vi "Logger.vi"(3 "Error In":errorcluster, 4 "Pipeline In":refnum<queue>, 5 "Logger Queue In":refnum<queue>) -> (0 "Error Out":errorcluster)   [LabVIEW 2016]
uses:
  Message Format.ctl
  StateDef_logger.ctl
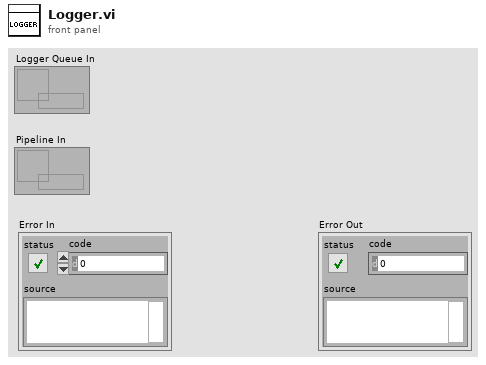
[diagram p1: front panel]
types:
  T1 = typedef "StateDef_Logger.ctl" = enum16{"Idle", "Open File", "Write to File", "Close File", "Exit"}
  T2 = enum16{"open", "open or create", "create or replace", "create", "open (read-only)"}
  T3 = typedef "Message Format.ctl" = cluster{"header":string, "data":variant}
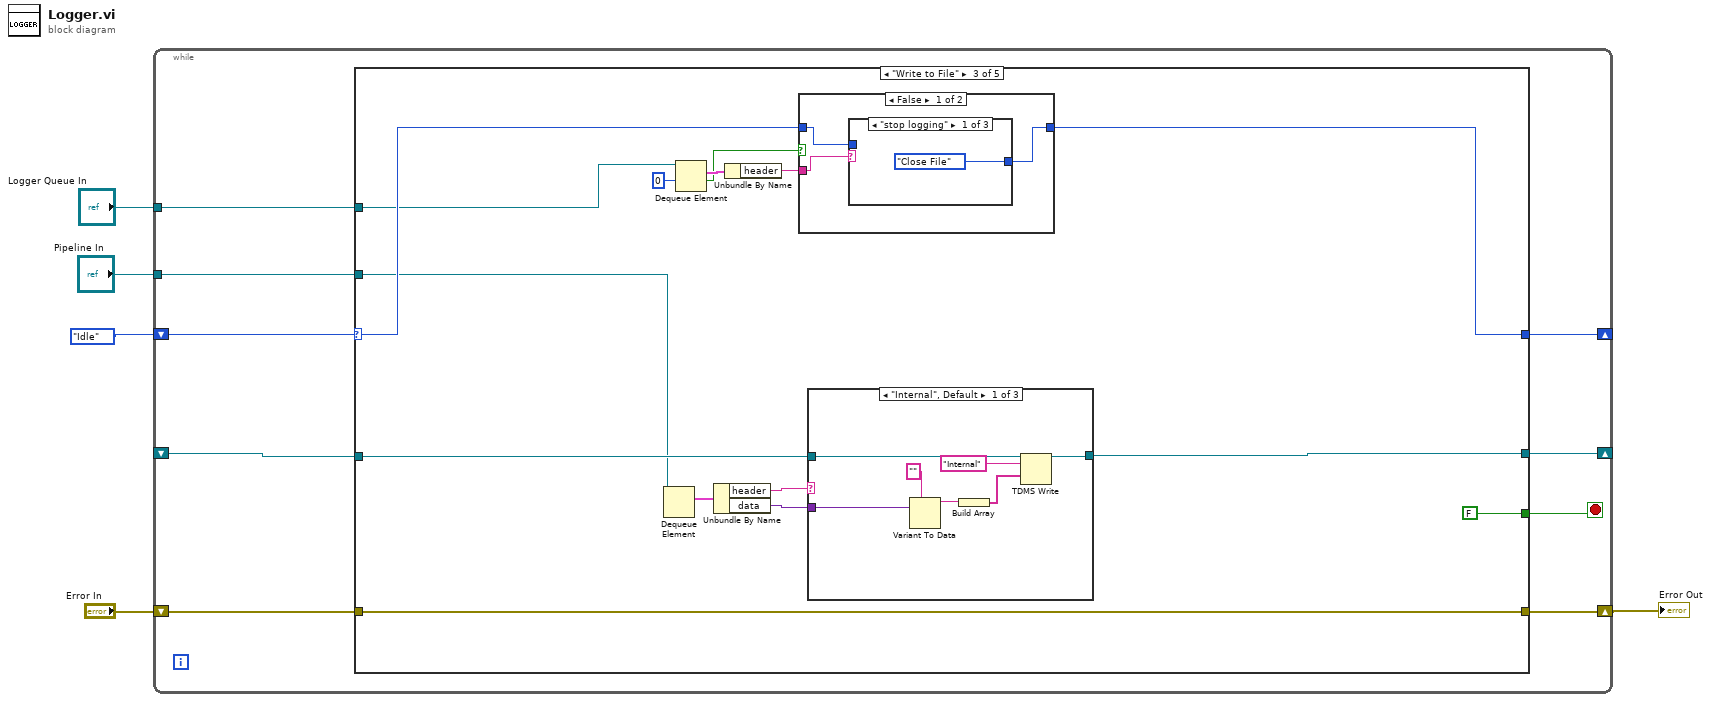
[diagram p0: block diagram]
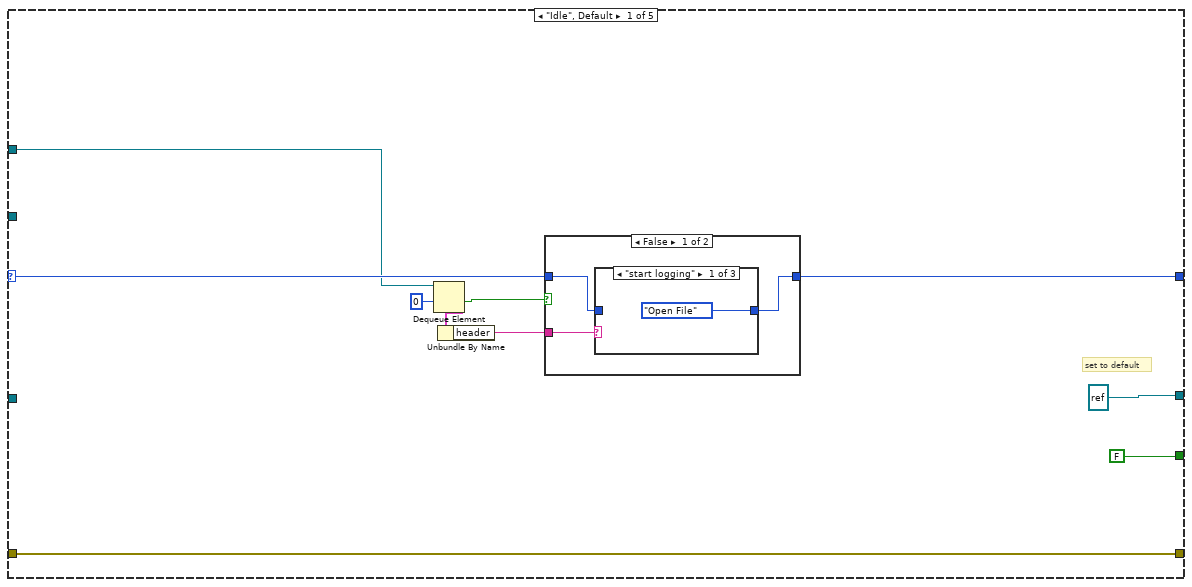
[diagram p2: hidden frame]
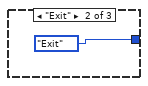
[diagram p3: hidden frame]
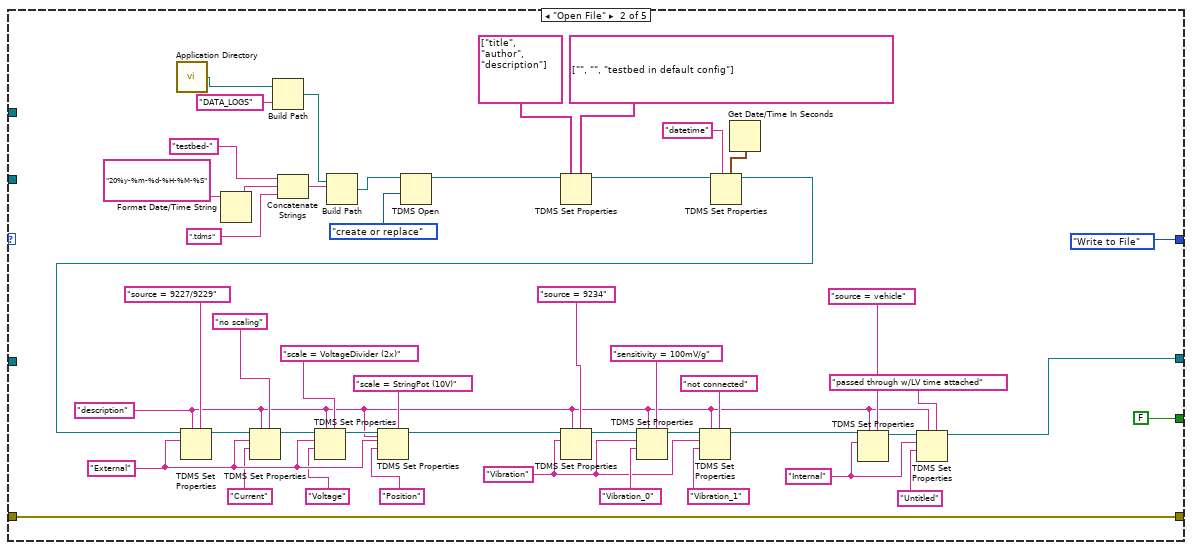
[diagram p6: hidden frame]
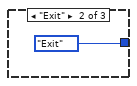
[diagram p7: hidden frame]
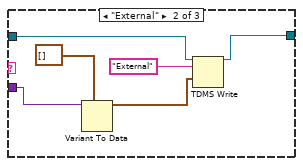
[diagram p10: hidden frame]
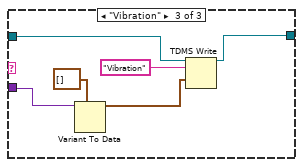
[diagram p11: hidden frame]
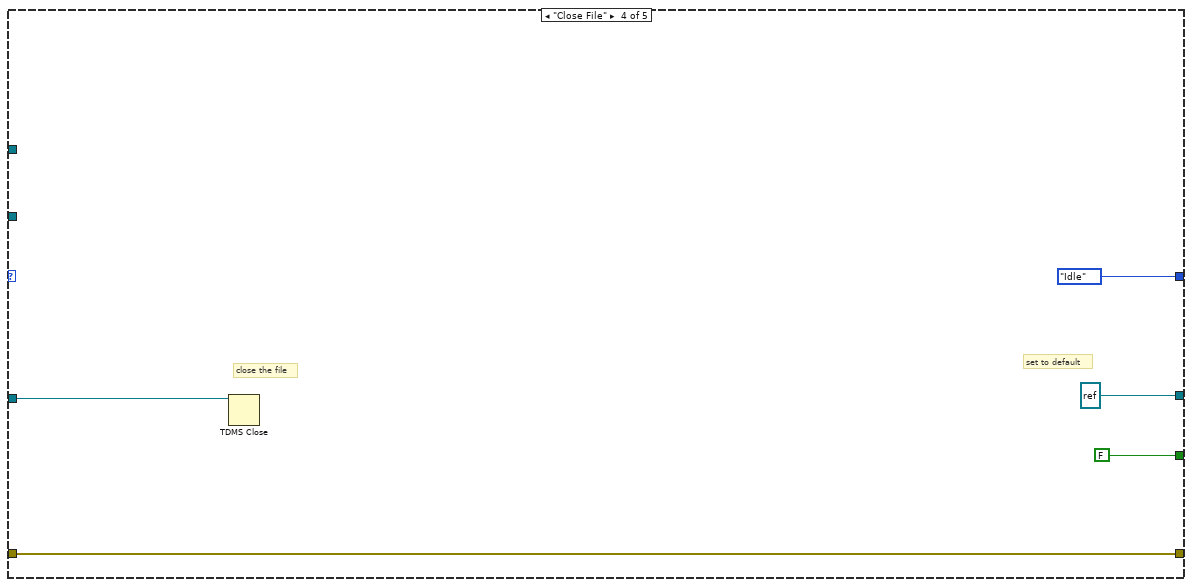
[diagram p12: hidden frame]
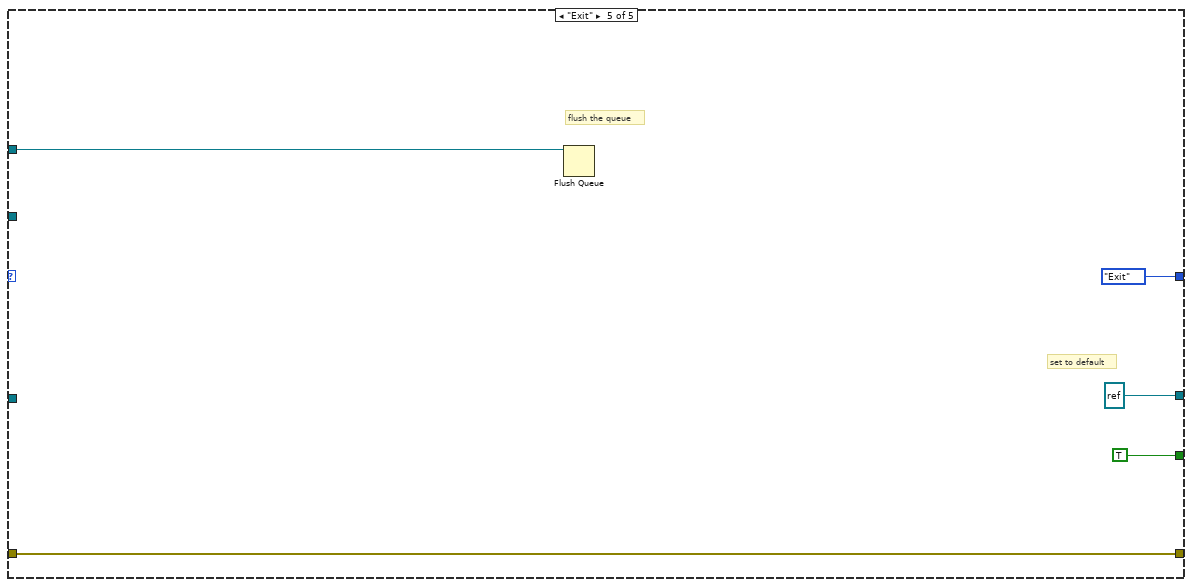
[diagram p13: hidden frame]
diagram:
  n1 = while {
    shift-right: [w11] -> _
    shift-left: StateDef_Logger."Idle" -> [w12]
    shift-right: [w14] -> _
    shift-left: _ -> [w13]
    tunnel: "Logger Queue In" -> [w8]
    tunnel: "Pipeline In" -> [w9]
    shift-right: [w7] -> w1
    shift-left: "Error In" -> [w6]
    stop <- w10 stop-if-true
    n2 = case shown="\"Write to File\"" w12 {
      selector: w12 -> [w24 _ w89 _ _]
      tunnel: [refnum<k34> refnum ("tdms file out") w38 w94 refnum<k34> refnum ("tdms file default") refnum<k34> refnum ("tdms file default")] -> w14
      tunnel: w13 -> [_ _ w93 w123 _]
      tunnel: [w23 StateDef_Logger."Write to File" w88 StateDef_Logger."Idle" StateDef_Logger."Exit"] -> w11
      tunnel: [FALSE FALSE FALSE FALSE TRUE] -> w10
      tunnel: w9 -> [_ _ w82 _ _]
      tunnel: w8 -> [w17 _ w83 _ w127]
      tunnel: [w16 w32 w80 w121 w126] -> w7
      tunnel: w6 -> [w16 w32 w80 w121 w126]
      frame "Idle", Default {
        # "set to default"
        n3 = Dequeue Element(queue=w17, timeout in ms (-1)=0) -> (element=w21:T3, timed out?=w19:bool)  [unwired: 1 in, 2 out]
        n4 = Unbundle By Name(w21) -> ("header"=w18:string)
        n5 = case shown="False" w19 {
          tunnel: w24 -> [w26 w31]
          tunnel: [w27 w31] -> w23
          tunnel: w18 -> [w25 _]
          frame False {
            n6 = case shown="\"start logging\"" w25 {
              tunnel: [StateDef_Logger."Open File" StateDef_Logger."Exit" w30] -> w27
              tunnel: w26 -> [_ _ w30]
              frame "start logging" {
              }
              frame "Exit" {
              }
              frame "any other", Default {
              }
            }
          }
          frame True {
            # "no pending msg if time out -> pass the state through"
          }
        }
      }
      frame "Open File" {
        w40 = "Internal" ("group name")
        w47 = "Vibration" ("group name")
        w39 = "description" ("group name")
        w65 = "External" ("group name")
        n7 = call <vilib>:"Application Directory.vi"() -> ("Application Directory"=w36:path)
        n8 = Format Date/Time String(time format string (%c)="20%y-%m-%d-%H-%M-%S") -> (date/time string=w76:string)  [unwired: 2 in]
        n9 = Build Path(base path=w36, name or relative path="DATA_LOGS") -> (appended path=w34:path)
        n10 = Concatenate Strings("testbed-" ("Data type"), w76, ".tdms") -> (w79:string)
        n11 = Build Path(base path=w34, name or relative path=w79) -> (appended path=w74:path)
        n12 = TDMS Open(10:T2."create or replace" ("operation (0:open)"), 11:w74) -> (3:w66:refnum<k34>)  [unwired: 5 in, 1 out]
        n13 = TDMS Set Properties(5:string[] ["", "", "testbed in default config"] ("property values"), 7:string[] ["title", "author", "description"] ("property names"), 11:w66) -> (3:w68:refnum<k34>)  [unwired: 3 in, 3 out]
        n14 = Get Date/Time In Seconds() -> (seconds since 1Jan1904=w69:timestamp)
        n15 = TDMS Set Properties(5:w69, 7:"datetime" ("Title"), 11:w68) -> (3:w67:refnum<k34>)  [unwired: 3 in, 3 out]
        n16 = TDMS Set Properties(5:"source = 9227/9229" ("group name"), 7:w39, 10:w65, 11:w67) -> (3:w64:refnum<k34>)  [unwired: 2 in, 3 out]
        n17 = TDMS Set Properties(5:"no scaling" ("group name"), 7:w39, 9:"Current" ("channel name"), 10:w65, 11:w64) -> (3:w63:refnum<k34>)  [unwired: 1 in, 3 out]
        n18 = TDMS Set Properties(5:"scale = VoltageDivider (2x)" ("group name"), 7:w39, 9:"Voltage" ("channel name"), 10:w65, 11:w63) -> (3:w62:refnum<k34>)  [unwired: 1 in, 3 out]
        n19 = TDMS Set Properties(5:"scale = StringPot (10V)" ("group name"), 7:w39, 9:"Position" ("channel name"), 10:w65, 11:w62) -> (3:w54:refnum<k34>)  [unwired: 1 in, 3 out]
        n20 = TDMS Set Properties(5:"source = 9234" ("group name"), 7:w39, 10:w47, 11:w54) -> (3:w46:refnum<k34>)  [unwired: 2 in, 3 out]
        n21 = TDMS Set Properties(5:"sensitivity = 100mV/g" ("group name"), 7:w39, 9:"Vibration_0" ("channel name"), 10:w47, 11:w46) -> (3:w49:refnum<k34>)  [unwired: 1 in, 3 out]
        n22 = TDMS Set Properties(5:"not connected" ("group name"), 7:w39, 9:"Vibration_1" ("channel name"), 10:w47, 11:w49) -> (3:w45:refnum<k34>)  [unwired: 1 in, 3 out]
        n23 = TDMS Set Properties(5:"source = vehicle" ("group name"), 7:w39, 10:w40, 11:w45) -> (3:w41:refnum<k34>)  [unwired: 2 in, 3 out]
        n24 = TDMS Set Properties(5:"passed through w/LV time attached" ("group name"), 7:w39, 9:"Untitled" ("channel name"), 10:w40, 11:w41) -> (3:w38:refnum<k34>)  [unwired: 1 in, 3 out]
      }
      frame "Write to File" {
        n25 = Dequeue Element(queue=w82) -> (element=w92:T3)  [unwired: 2 in, 3 out]
        n26 = Dequeue Element(queue=w83, timeout in ms (-1)=0) -> (element=w87:T3, timed out?=w84:bool)  [unwired: 1 in, 2 out]
        n27 = Unbundle By Name(w92) -> ("header"=w91:string, "data"=w90:variant)
        n28 = Unbundle By Name(w87) -> ("header"=w85:string)
        n29 = case shown="False" w84 {
          tunnel: w89 -> [w96 w101]
          tunnel: [w97 w101] -> w88
          tunnel: w85 -> [w95 _]
          frame False {
            n30 = case shown="\"stop logging\"" w95 {
              tunnel: [StateDef_Logger."Close File" StateDef_Logger."Exit" w100] -> w97
              tunnel: w96 -> [_ _ w100]
              frame "stop logging" {
              }
              frame "Exit" {
              }
              frame "any other", Default {
              }
            }
          }
          frame True {
            # "no pending msg if time out -> pass the state through"
          }
        }
        n31 = case shown="\"Internal\", Default" w91 {
          tunnel: w93 -> [w106 w114 w118]
          tunnel: w90 -> [w107 w112 w117]
          tunnel: [w105 w110 w116] -> w94
          frame "Internal", Default {
            n32 = Variant To Data(type="", Variant=w107) -> (data=w103:string)  [unwired: 1 in, 1 out]
            n33 = Build Array(w103) -> (w102:string[])
            n34 = TDMS Write(0:w106, 5:"Internal" ("group name in (Untitled)"), 9:w102) -> (4:w105:refnum<k34>)  [unwired: 3 in, 3 out]
          }
          frame "External" {
            n35 = Variant To Data(type=waveform(dbl)[] [] ("data"), Variant=w112) -> (data=w111:waveform(dbl)[])  [unwired: 1 in, 1 out]
            n36 = TDMS Write(0:w114, 5:"External" ("group name in (Untitled)"), 9:w111) -> (4:w110:refnum<k34>)  [unwired: 3 in, 3 out]
          }
          frame "Vibration" {
            n37 = Variant To Data(type=waveform(dbl)[] [] ("data"), Variant=w117) -> (data=w119:waveform(dbl)[])  [unwired: 1 in, 1 out]
            n38 = TDMS Write(0:w118, 5:"Vibration" ("group name in (Untitled)"), 9:w119) -> (4:w116:refnum<k34>)  [unwired: 3 in, 3 out]
          }
        }
      }
      frame "Close File" {
        # "close the file"
        # "set to default"
        n39 = TDMS Close(11:w123) -> ()  [unwired: 1 in, 2 out]
      }
      frame "Exit" {
        # "flush the queue"
        # "set to default"
        n40 = Flush Queue(queue=w127) -> ()  [unwired: 1 in, 3 out]
      }
    }
  }
  "Error Out" <- w1
